vi "Initialize.vi"(8 "error in (no error)":errorcluster, 11 "Transfer User Interface in":refnum<class "Transfer User Interface.lvclass">) -> (0 "error out":errorcluster, 3 "Transfer User Interface out":refnum<class "Transfer User Interface.lvclass">)   [LabVIEW 2017, in "GE Reflective Memory.lvlib" / "Transfer User Interface.lvclass"]
uses:
  Transfer User Interface.lvclass
  Configurations/Transfer/Transfer Configuration.lvclass
  DSF Core.lvlibp/Classes/User Interface/User Interface.lvclass
  C:/Git/DSF/Components/DSF Core.lvlibp/Classes/Configuration/Configuration.lvclass
  C:/Git/DSF/Components/DSF Core.lvlibp/Classes/User Interface/User Interface.lvclass
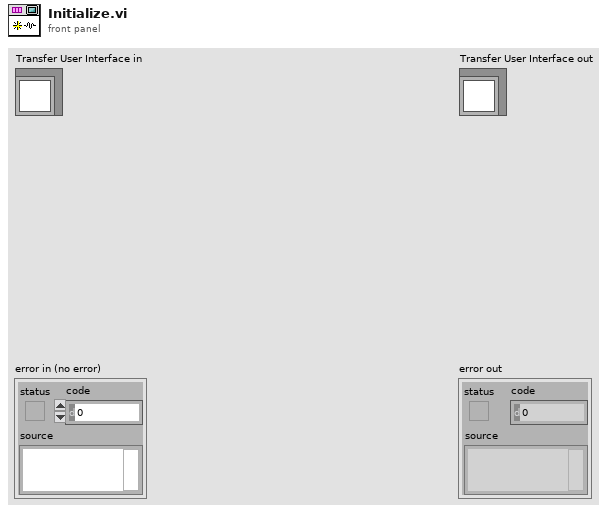
[diagram p1: front panel]
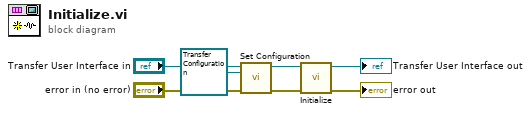
[diagram p0: block diagram]
diagram:
  n1 = call "Set Configuration.vi"("error in (no error)"="error in (no error)", "configuration"=refnum<class "Transfer Configuration.lvclass"> refnum ("GE Reflective Memory.lvlib:Transfer Configuration.lvclass"), "User Interface in"="Transfer User Interface in") -> ("error out"=w2:errorcluster, "User Interface out"=w3:refnum<class "Transfer User Interface.lvclass">)  [unwired: 7 in]
  n2 = call-parent "Initialize.vi"("error in (no error)"=w2, "User Interface in"=w3) -> ("error out"=→"error out":errorcluster, "User Interface out"=→"Transfer User Interface out":refnum<class "Transfer User Interface.lvclass">)  [unwired: 8 in]
